vi "Pneumatics Begin.vi"(8 "error in (no error)":errorcluster, 10 "Data Out":variant, 11 "Pneumatics in":refnum<class "Pneumatics.lvclass">) -> (0 "error out":errorcluster, 3 "Pneumatics out":refnum<class "Pneumatics.lvclass">)   [LabVIEW 2019]
doc: "This VI initializes the pneumatics using the config file class and the configuration variant.\nThis VI does not live inside the pneumatics library because it depends on the config file class."
uses:
  Classes/Pnematics control/Pneumatics.lvclass
  Classes/Pnematics control/Solenoids/Solenoids.lvclass
  Classes/Configuration File/Configuration File.lvclass
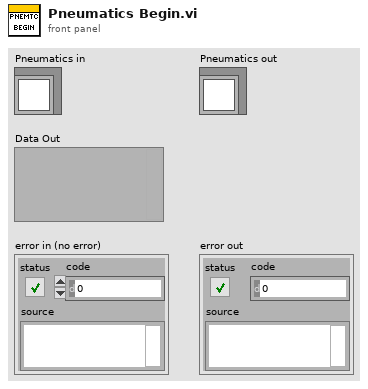
[diagram p1: front panel]
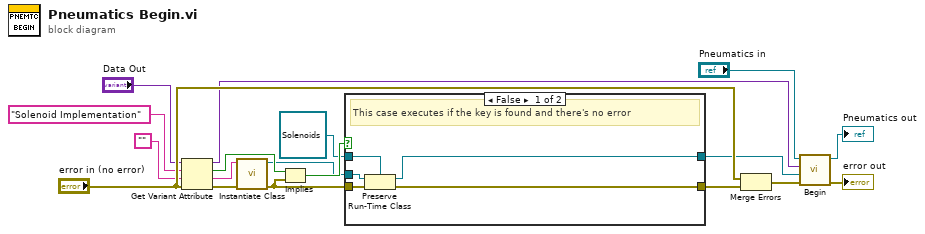
[diagram p0: block diagram]
diagram:
  n1 = Get Variant Attribute(Variant="Data Out", name="Solenoid Implementation", default value (empty Variant)="", error in="error in (no error)") -> (duplicate Variant=w12:variant, found=w8:bool, value=w4:string, error out=w3:errorcluster)
  n2 = call "Instantiate Class.vi"("error in (no error)"=w3, "String"=w4) -> ("error out"=w10:errorcluster, "LabVIEW Object out"=w6:refnum<class>)  [unwired: 8 in]
  n3 = Implies(1:w10, 2:w8) -> (0:w9:bool)
  n4 = case shown="False" w9 {
    tunnel: w10 -> [w23 w25]
    tunnel: [w22 w25] -> w5
    tunnel: w6 -> [w21 _]
    tunnel: refnum<class "Solenoids.lvclass"> refnum ("s? t:f") -> [w20 w24]
    tunnel: [w19 w24] -> w13
    frame False {
      # "This case executes if the key is found and there's no error"
      n5 = Preserve Run-Time Class(object in=w21, error in=w23, 2:w20) -> (object out=w19:refnum<class "Solenoids.lvclass">, error out=w22:errorcluster)
    }
    frame True {
      # "The key wasn't found of there's an error"
    }
  }
  n6 = Merge Errors("error in (no error)", w5) -> (w11:errorcluster)
  n7 = call-dynamic "Begin.vi"("error in (no error)"=w11, "Pneumatics control.lvlib:Solenoids.lvclass"=w13, "Settings"=w12, "Pneumatics in"="Pneumatics in") -> ("error out"=→"error out":errorcluster, "Pneumatics out"=→"Pneumatics out":refnum<class "Pneumatics.lvclass">)  [unwired: 6 in]
